vi "SMC Get Message.vi"(0 "Timeout (ms)":i32) -> (1 "SMC Message Type":T1(ring)=enum."Ping=", 2 "Text":string)   [LabVIEW 2019]
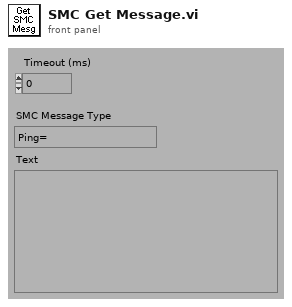
[diagram p1: front panel]
types:
  T1 = enum16{"Bad Message", "DoNothing", "Read=", "GenEvent=", "MagStatus=", "Control", "Setpoint=", "Setrate=", "Heater=", "Ping=", "Stop", "Beep"}
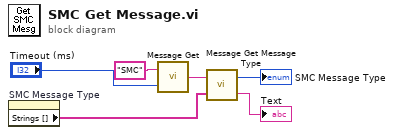
[diagram p0: block diagram]
diagram:
  n1 = property on="SMC Message Type" class="Enum (strict)"() -> ("Strings []"=w3:string[])  [unwired: 2 in, 2 out]
  n2 = call "Message Get.vi"("Timeout ms (-1)"="Timeout (ms)", "Module"="SMC") -> ("data out"=w5:string)
  n3 = call "Message Get Message Type.vi"("Message Types"=w3, "Message"=w5) -> ("Trailing text"=→"Text":string, "Message Type"=→"SMC Message Type":i32)
